vi "Delaunay Triangulation.vi"(10 "Y":dbl[](array[numeric]), 11 "X":dbl[](array[numeric])) -> (0 "error":i32, 3 "Triangles":i32[][](array[numeric]))   [LabVIEW 2017, in "NI_AAL_Geometry.lvlib"]
doc: "Computes the Delaunay triangulation of the specified points in the plane."
uses:
  <vilib>/Analysis/NI_AAL_Geometry.lvlib
  <vilib>/Analysis/geometry.llb/DT_Output Option.ctl
panel:
  # "Delaunay Triangulation"
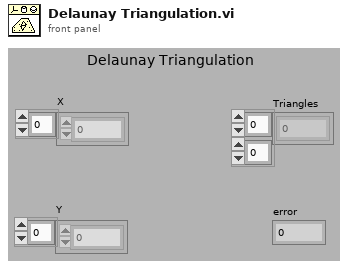
[diagram p1: front panel]
types:
  T1 = typedef "NI_AAL_Geometry.lvlib/DT_Output Option.ctl" = i32
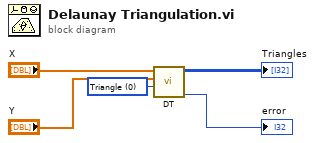
[diagram p0: block diagram]
diagram:
  w1 = T1 0 items=["Triangle", "Adj Triangle", "Segment"] ("output option")
  n1 = call <vilib>:"DT.vi"("output option"=w1, "Y"="Y", "X"="X") -> ("error"=→"error":i32, "Triangles"=→"Triangles":i32[][])  [unwired: 7 in]
